vi "Verify Information.vi"(2 "Password":string, 3 "User Name":string) -> (0 "Access Granted":bool, 1 "Operator":string)   [LabVIEW 2014]
panel:
  in  "Table":string[][](table)=[["Administrador", "1234"], ["Entrenador", "5678"], ["alpineda", "7875"]]
  # "Employee Name"
  # "Password"
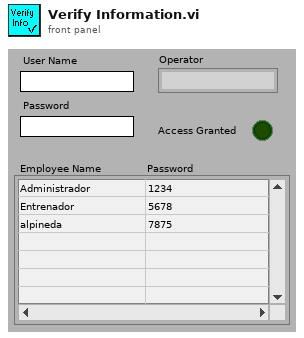
[diagram p1: front panel]
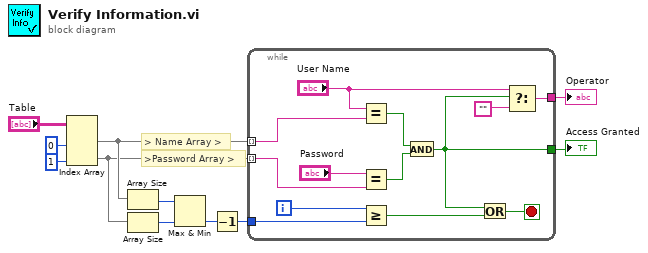
[diagram p0: block diagram]
diagram:
  # ">Password Array >"
  # "> Name Array >"
  n1 = Index Array "Index Array"(array="Table", index (col) #1=0 ("disabled index (col)"), index (col) #2=1 ("index (col)")) -> (element #1=w6:string[], element #2=w5:string[])  [unwired: 2 in]
  n2 = Array Size(array=w6) -> (size(s)=w3:i32)
  n3 = Array Size(array=w5) -> (size(s)=w2:i32)
  n4 = Max & Min(x=w3, y=w2) -> (min(x,y)=w4:i32)  [unwired: 1 out]
  n5 = Decrement(x=w4) -> (x-1=w11:i32)
  n6 = while {
    tunnel: w11 -> [w22]
    tunnel: [w15] -> w10
    tunnel: w6 -> [w14] mode=indexing
    tunnel: w5 -> [w13] mode=indexing
    tunnel: [w12] -> w1
    i -> [w21]
    stop <- w19 stop-if-true
    n7 = Equal?(x="User Name", y=w14) -> (x = y?=w24:bool)
    n8 = Equal?(x="Password", y=w13) -> (x = y?=w23:bool)
    n9 = Greater Or Equal?(x=w21, y=w22) -> (x >= y?=w20:bool)
    n10 = And(x=w24, y=w23) -> (x .and. y?=w12:bool)
    n11 = Or(x=w12, y=w20) -> (x .or. y?=w19:bool)
    n12 = Select(t="User Name", s=w12, f="") -> (s? t:f=w15:string)
  }
  "Operator" <- w10
  "Access Granted" <- w1
